vi "Required Font Scale.vi"(4 "Thickness (Default: 1)":i32=1, 5 "OpenCV Font Face":T1, 8 "error in (no error)":errorcluster, 11 "Required Text Height":u16) -> (0 "error out":errorcluster, 3 "Font Scale":dbl)   [LabVIEW 2020, in "image.lvlib"]
uses:
  image.lvlib
  Font Face.ctl
  common/common.lvlib
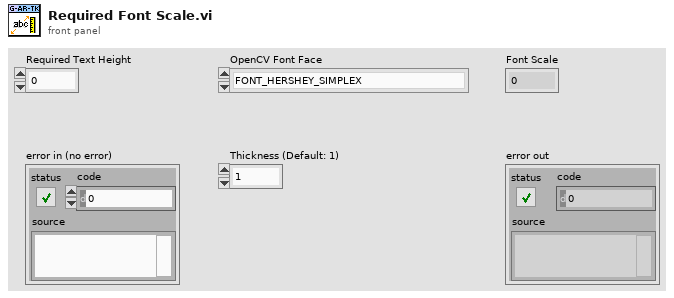
[diagram p1: front panel]
types:
  T1 = typedef "image.lvlib/Font Face.ctl" = enum8{"FONT_HERSHEY_SIMPLEX", "FONT_HERSHEY_PLAIN", "FONT_HERSHEY_DUPLEX", "FONT_HERSHEY_COMPLEX", "FONT_HERSHEY_TRIPLEX", "FONT_HERSHEY_COMPLEX_SMALL", "FONT_HERSHEY_SCRIPT_SIMPLEX", "FONT_HERSHEY_SCRIPT_COMPLEX", "FONT_ITALIC"}
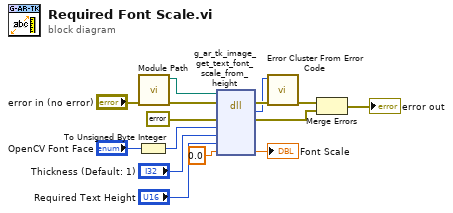
[diagram p0: block diagram]
diagram:
  n1 = To Unsigned Byte Integer(number="OpenCV Font Face") -> (unsigned 8bit integer=w12:u8)
  n2 = call "Module Path.vi"("error in (no error)"="error in (no error)") -> ("error out"=w2:errorcluster, "Path"=w1:path)  [unwired: 9 in]
  n3 = dll-call lib="?" fn="g_ar_tk_image_get_text_font_scale_from_height"(path in=w1, error in=w2, "error_cluster"=errorcluster {"status"=FALSE, "code"=0, "source"=""} ("error constant"), "font_face"=w12, "thickness"="Thickness (Default: 1)", "Required Height"="Required Text Height", "Font Scale"=0.0) -> (error out=w11:errorcluster, "MgErr"=w10:i32, "error_cluster"=w7:errorcluster, "Font Scale"=→"Font Scale":dbl)  [unwired: 4 in, 1 out]
  n4 = call <vilib>:"Error Cluster From Error Code.vi"("error in (no error)"=w11, "error code (0)"=w10) -> ("error out"=w9:errorcluster)  [unwired: 7 in]
  n5 = Merge Errors(w9, w7) -> (→"error out":errorcluster)
